vi "Hatch Controller.vi"(8 "error in":errorcluster) -> ()   [LabVIEW 2019]
doc: "This VI executes continuously carrying out the current operation and responding to updates or new operations. It will often contain the timing or control code that is difficult to place directly in TeleOp. This VI generally opens all sensors and motors and isolates the rest of the robot code from knowing how the operations are carried out."
uses:
  <vilib>/Rock Robotics/WPI/Framework/Completion Status.ctl
  Hatch Setpoints.ctl
  Hatch Operations.ctl
  <vilib>/Rock Robotics/WPI/Solenoid/WPI_SolenoidValue.ctl
  <vilib>/Rock Robotics/WPI/Solenoid/WPI_SolenoidSetEnum.vi
  <vilib>/Rock Robotics/Network Tables/NT Write Boolean.vi
panel:
  in  "Interactive Values":T1
  out "Current\nCmd":string
  in  "Buttons":cluster{"Execute Cmd":bool, "Abort Cmd":bool}
  out "Command Timing":cluster{"Start Time (ms)":u32, "Iterations":i32}
  out "Status":T4
  # "Tip: It may be helpful to observe inputs and sensor values.\nYou may also want to display tuning or debugging controls."
  # "Interactive Command: You may fill in the settings for a command\nand schedule it with the Execute button. You can observe and abort\nany command while fine tuning the code for the controller."
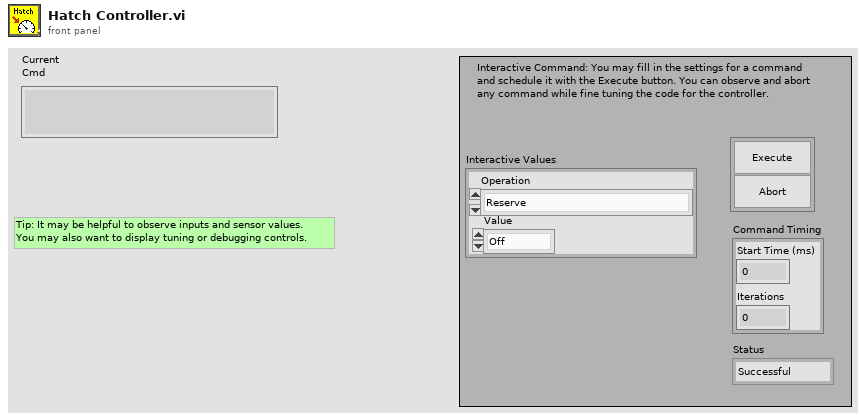
[diagram p1: front panel]
types:
  T1 = typedef "Hatch Setpoints.ctl" = cluster{"Operation":T2, "Relay Value":T3}
  T2 = typedef "Hatch Operations.ctl" = enum16{"Reserve", "Read Current", "Immediate"}
  T3 = typedef "WPI_SolenoidValue.ctl" = enum16{"Off", "On", "Forward", "Reverse"}
  T4 = typedef "Completion Status.ctl" = enum16{"Successful", "Aborted", "Incomplete"}
  T5 = typedef "WPI_SolenoidDevRef.ctl" = cluster{"DevStatus":errorcluster, "Pneumatics Control Module":u8, "Forward Solenoid Channel":T6, "Reverse Solenoid Channel":T6}
  T6 = typedef "WPI_SolenoidChannel.ctl" = enum8{"Solenoid 0", "Solenoid 1", "Solenoid 2", "Solenoid 3", "Solenoid 4", "Solenoid 5", "Solenoid 6", "Solenoid 7", "Invalid"}
  T7 = typedef "Command Status Info.ctl" = cluster{"Name":string, "Status":T4, "notifier out":T8}
  T8 = typedef "Completion Notifier.ctl" = refnum<notifier>
  T9 = cluster{"Current Command":T1, "Command Timing":cluster{"Start Time (ms)":u32, "Iterations":i32}, "Command Arguments":cluster{"Command Info":T7, "Description":string, "Default Command":T1, "queue out":refnum<queue>, "Subsystem Name":string}}
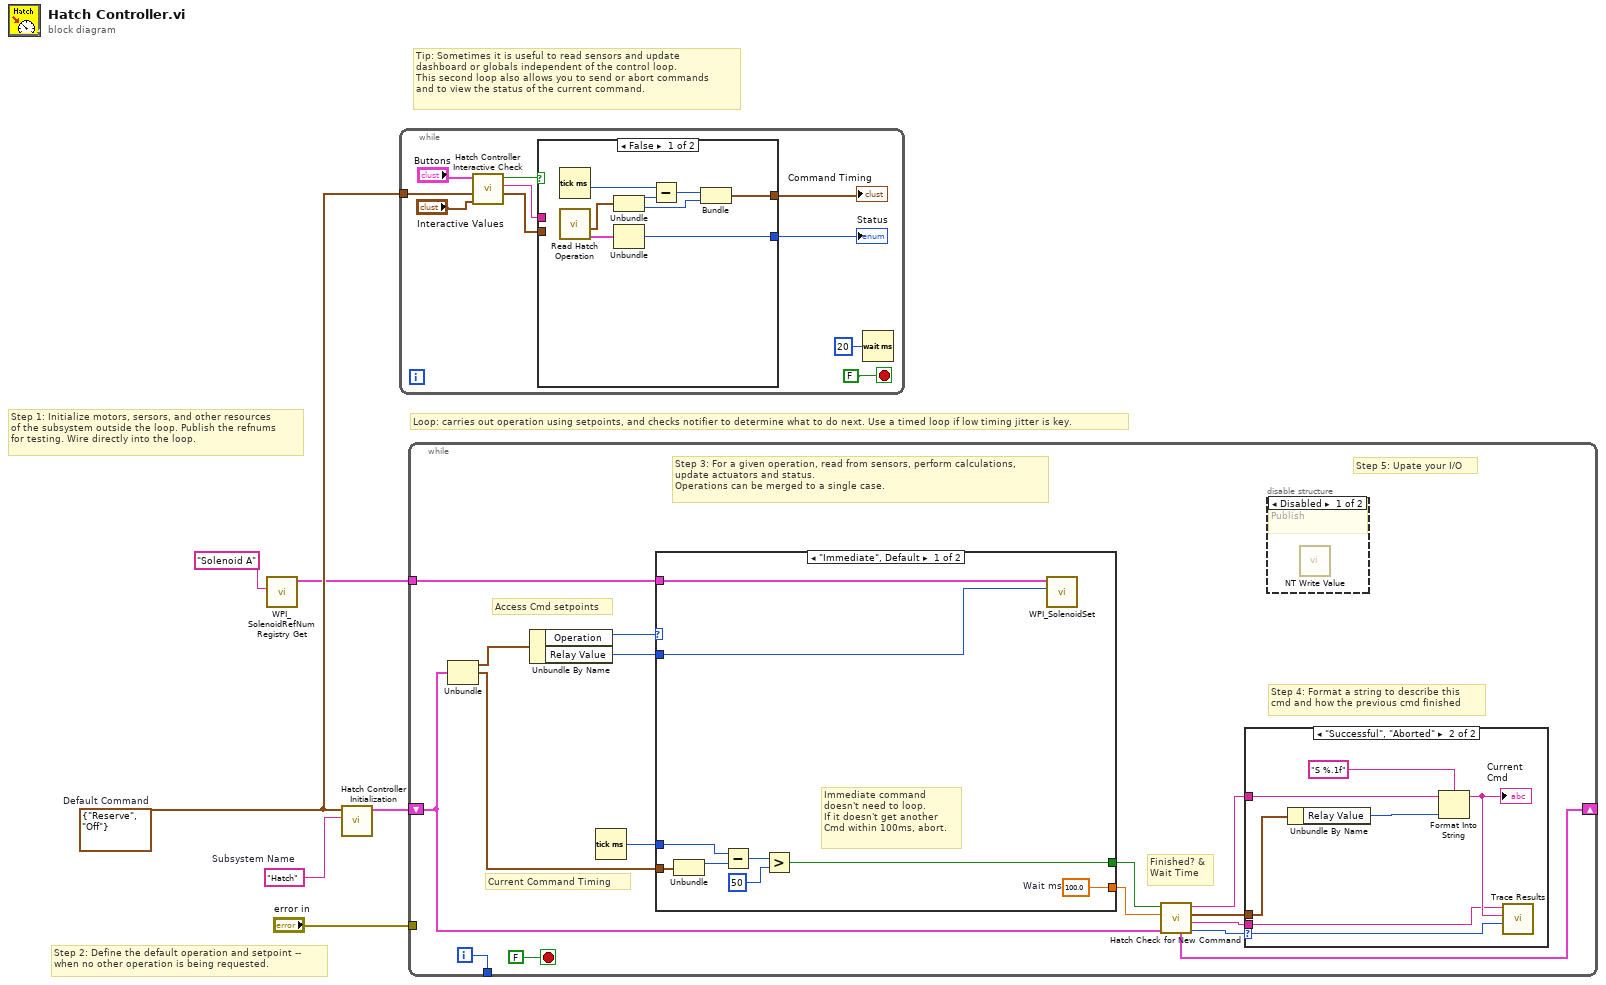
[diagram p0: block diagram]
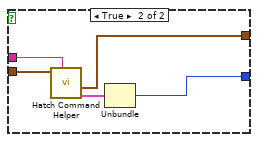
[diagram p2: hidden frame]
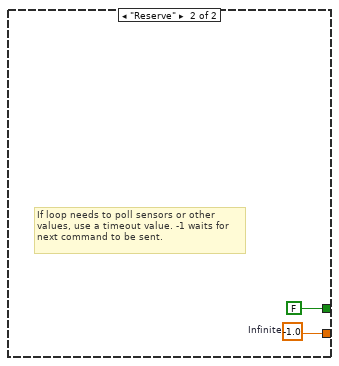
[diagram p5: hidden frame]
diagram:
  w3 = T1 {"Operation"=enum."Reserve", "Relay Value"=enum."Off"}  # Default Command
  w4 = "Hatch"  # Subsystem Name
  # "Tip: Sometimes it is useful to read sensors and update\ndashboard or globals independent of the control loop.\nThis second loop also allows you to send or abort commands\nand to view the status of the current command."
  # "Step 2: Define the default operation and setpoint --\nwhen no other operation is being requested."
  # "Step 1: Initialize motors, sersors, and other resources\nof the subsystem outside the loop. Publish the refnums\nfor testing. Wire directly into the loop."
  # "Loop: carries out operation using setpoints, and checks notifier to determine what to do next. Use a timed loop if low timing jitter is key."
  n1 = call <vilib>:"WPI_SolenoidRefNum Registry Get.vi"("refnum name"="Solenoid A") -> ("SolenoidDevRef"=w1:T5)  [unwired: 9 in, 1 out]
  n2 = call "Hatch Controller Initialization.vi"("Subsystem Name"=w4, "Default Command"=w3) -> ("Current Command"=w5:T9)  [unwired: 9 in]
  n3 = while {
    tunnel: w3 -> [w13]
    stop <- FALSE stop-if-true
    n4 = call "Hatch Controller Interactive Check.vi"("Interactive Command in"="Interactive Values", "Default Command"=w13, "Buttons"="Buttons") -> ("Interactive Command out"=w10:T1, "Trace String"=w11:string, "Schedule"=w12:bool)  [unwired: 6 in]
    n5 = case shown="False" w12 {
      tunnel: [w24 w29] -> w9
      tunnel: w10 -> [_ w27]
      tunnel: [w20 w25] -> w8
      tunnel: w11 -> [_ w28]
      frame False {
        n6 = Tick Count (ms)() -> (millisecond timer value=w19:u32)
        n7 = call "Read Hatch Operation.vi"() -> ("Command Info"=w17:T7, "SubSystem Data"=w18:T1)  [unwired: 9 in, 1 out]
        n8 = Unbundle(w18) -> ("Operation"=w23:T2, "Relay Value"=w21:T3)
        n9 = Unbundle(w17) -> ("Status"=w24:T4)  [unwired: 2 out]
        n10 = Subtract(x=w19, y=w23) -> (x-y=w22:u32)
        n11 = Bundle(w22, "Relay Value"=w21) -> (w20:cluster{u32, "Relay Value":T3})  [unwired: 1 in]
      }
      frame True {
        n12 = call "Hatch Command Helper.vi"("Description"=w28, "SubSystem Data"=w27) -> ("Command Info Out"=w26:T7, "Command Timing"=w25:cluster{"Start Time (ms)":u32, "Iterations":i32})  [unwired: 7 in, 1 out]
        n13 = Unbundle(w26) -> ("Status"=w29:T4)  [unwired: 2 out]
      }
    }
    "Status" <- w9
    "Command Timing" <- w8
    n14 = Wait (ms)(milliseconds to wait=u32 20) -> ()  [unwired: 1 out]
  }
  n15 = while {
    shift-right: [w38] -> _
    shift-left: w5 -> [w31]
    tunnel: [w44] -> _
    tunnel: "error in" -> [_]
    tunnel: w1 -> [w30]
    i -> [w44]
    stop <- FALSE stop-if-true
    # "Step 5: Upate your I/O"
    # "Step 4: Format a string to describe this\ncmd and how the previous cmd finished"
    # "Current Command Timing"
    # "Access Cmd setpoints"
    # "Finished? &\nWait Time"
    # "Step 3: For a given operation, read from sensors, perform calculations,\nupdate actuators and status.\nOperations can be merged to a single case."
    n16 = Unbundle(w31) -> ("Current Command"=w43:T1, "Command Timing"=w39:cluster{"Start Time (ms)":u32, "Iterations":i32})  [unwired: 1 out]
    n17 = Unbundle By Name(w43) -> ("Operation"=w42:T2, "Relay Value"=w41:T3)
    n18 = Tick Count (ms)() -> (millisecond timer value=w40:u32)
    n19 = case shown="\"Immediate\", Default" w42 {
      tunnel: [w61 w63] -> w36
      tunnel: [w55 FALSE ("ignore previous (F)")] -> w37
      tunnel: w39 -> [w57 _]
      tunnel: w41 -> [w53 _]
      tunnel: w40 -> [w56 _]
      tunnel: w30 -> [w54 _]
      frame "Immediate", Default {
        w61 = 100.0  # Wait ms
        # "Immediate command\ndoesn't need to loop.\nIf it doesn't get another\nCmd within 100ms, abort."
        n20 = Unbundle(w57) -> ("Start Time (ms)"=w60:u32)  [unwired: 1 out]
        n21 = Subtract(x=w56, y=w60) -> (x-y=w59:u32)
        n22 = Greater?(x=w59, y=u8 50 ("Left Motor")) -> (0:w55:bool)
        n23 = call-poly <vilib>:"WPI_SolenoidSet.vi"("Value"=w53, "SolenoidDevRef"=w54) -> ()  [unwired: 8 in, 2 out]
      }
      frame "Reserve" {
        w63 = -1.0  # Infinite
        # "If loop needs to poll sensors or other\nvalues, use a timeout value. -1 waits for\nnext command to be sent."
      }
    }
    n24 = call "Hatch Check for New Command.vi"("Current Command"=w31, "Wait time (ms)"=w36, "Finished?"=w37) -> ("Completion"=w32:T4, "Subsystem Name"=w33:string, "Current Command"=w34:T1, "Initial Trace String"=w35:string, "NextCommand"=w38:T9)  [unwired: 4 in]
    n25 = case shown="\"Successful\", \"Aborted\"" w32 {
      selector: w32 -> [_ w52]
      tunnel: w35 -> [_ w48]
      tunnel: w34 -> [_ w49]
      tunnel: w33 -> [_ w46]
      frame "Incomplete", Default {
        # "Continuing current command"
      }
      frame "Successful", "Aborted" {
        # "Report and setup for next command"
        n26 = Unbundle By Name(w49) -> ("Relay Value"=w51:T3)
        n27 = Format Into String(format string="S %.1f", initial string=w48, w51) -> (resulting string=w47:string)  [unwired: 1 in, 1 out]
        "Current\nCmd" <- w47
        n28 = call <vilib>:"Trace Results.vi"("Status of previous command"=w52, "Description"=w47, "Subsystem"=w46) -> ()  [unwired: 9 in]
      }
    }
    n29 = disable-structure shown="Disabled" {
      frame Disabled {
        # "Publish"
        n30 = call-poly <vilib>:"NT Write Value.vi"() -> ()  [unwired: 11 in, 1 out]
      }
      frame Enabled {
      }
    }
  }
